vi "air resistancevi.vi"(9 "air density":dbl, 10 "CdA":dbl, 11 "V^2":dbl) -> (3 "result":dbl)   [LabVIEW 2014]
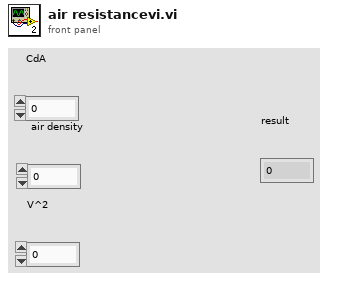
[diagram p1: front panel]
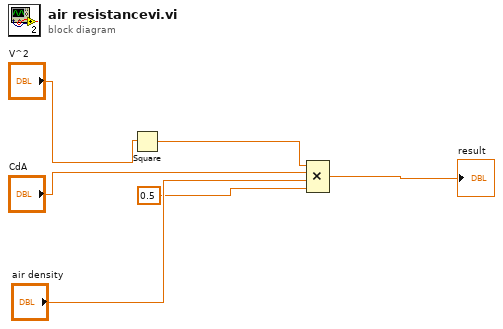
[diagram p0: block diagram]
diagram:
  n1 = Square(x="V^2") -> (x^2=w2:dbl)
  n2 = Compound Arithmetic op=MULTIPLY(w2, "CdA", "air density", 0.5 ("value")) -> (→"result":dbl)
